vi "Scan Chart View.vi"(10 "UserEvents in":refnum<class "UserEvents.lvclass">) -> ()   [LabVIEW 2015, in "FAMT Views.lvlib"]
uses:
  FAMT Views.lvlib
  UserEvents/UserEvents.lvclass
  UserEvents/UserEvents.lvclass/UserEvents.ctl
  Typedefs/State Types.ctl
  Typedefs/FAMT Typedefs.lvlib
panel:
  out "Chart":cluster{"Current Demand":dbl, dbl}(graph)
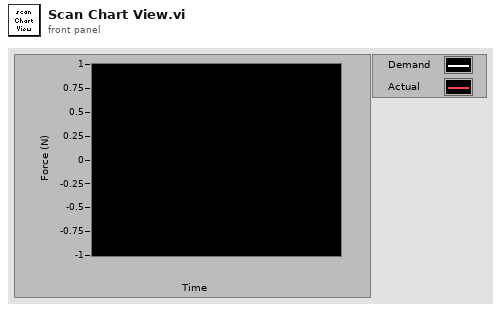
[diagram p1: front panel]
types:
  T1 = typedef "FAMT Typedefs.lvlib/Publish Data Events.ctl" = cluster{"State":refnum<user-event>, "ErrorCode":refnum<user-event>, "FC1 ILC Outputs":refnum<user-event>, "LogPath":refnum<user-event>, "FC1 ILC Inputs":refnum<user-event>, "Scan Progress":refnum<user-event>, "FC2 ILC Outputs":refnum<user-event>, "FC2 ILC Inputs":refnum<user-event>}
  T2 = cluster{"Event Registration Refnum":refnum<event-registration>, "Event Registration Refnum":refnum<event-registration>}
  T3 = typedef "FAMT Typedefs.lvlib/State Types.ctl" = enum16{"Offline State", "Fault State", "Standby State", "Disabled State", "Enabled State", "Wait For User Input State", "Perform Scan State"}
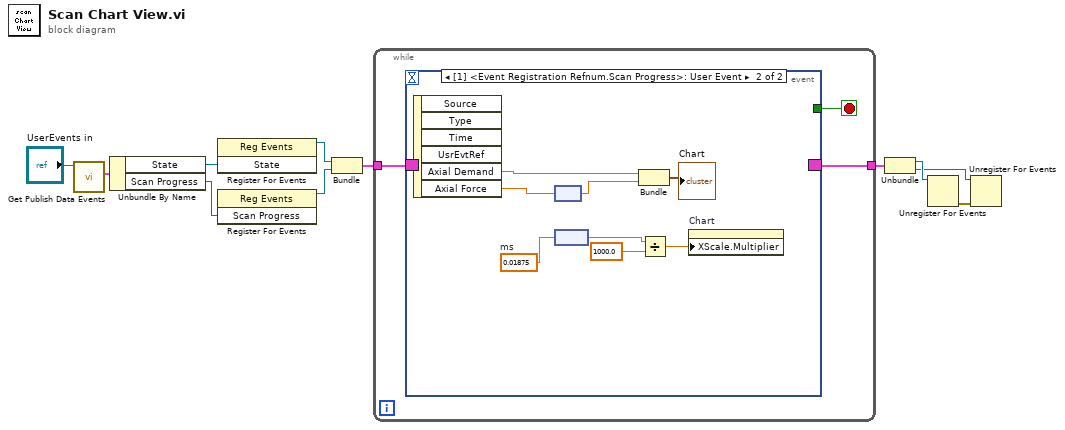
[diagram p0: block diagram]
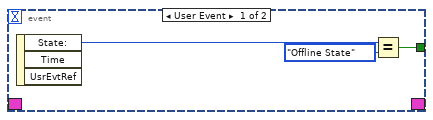
[diagram p2: hidden frame]
diagram:
  n1 = call "Get Publish Data Events.vi"("UserEvents in"="UserEvents in") -> ("Publish Data Events"=w8:T1)  [unwired: 9 in, 1 out]
  n2 = Unbundle By Name(w8) -> ("State"=w9:refnum<user-event>, "Scan Progress"=w7:refnum<user-event>)
  n3 = register-events(w9) -> (reference out=w11:refnum<event-registration>)  [unwired: 2 in, 1 out]
  n4 = register-events(w7) -> (reference out=w10:refnum<event-registration>)  [unwired: 2 in, 1 out]
  n5 = Bundle("Event Registration Refnum"=w11, "Event Registration Refnum"=w10) -> (w3:T2)  [unwired: 1 in]
  n6 = while {
    tunnel: w3 -> [w14]
    tunnel: [w13] -> w2
    stop <- w12 stop-if-true
    n7 = event shown="[1] <Event Registration Refnum.Scan Progress>: User Event" {
      selector: w14 -> [_ _]
      dyn-events: [_ _] -> w13
      timeout: _ -> [_ _]
      tunnel: [w16 _] -> w12
      event User Event {
        n8 = event-data() -> ("State:"=w15:T3)  [unwired: 1 in, 2 out]
        n9 = Equal?(x=w15, y=State_Types."Offline State") -> (x = y?=w16:bool)
      }
      event User Event {
        w19 = dbl[unit] 0.01875  # ms
        n10 = event-data() -> ("Axial Demand"=w20:dbl, "Axial Force"=w25:dbl[unit])  [unwired: 1 in, 4 out]
        n11 = node(w25) -> (w24:dbl)
        n12 = node(w19) -> (w22:dbl)
        n13 = Bundle("Axial Demand"=w20, w24) -> (→"Chart":cluster{"Axial Demand":dbl, dbl})  [unwired: 1 in]
        n14 = Divide(x=w22, y=1000.0) -> (x/y=w21:dbl)
        n15 = property on="Chart" class="WFChart (strict)"("XScale.Multiplier"=w21) -> ()  [unwired: 2 in, 2 out]
      }
    }
  }
  n16 = Unbundle(w2) -> ("Event Registration Refnum"=w6:refnum<event-registration>, "Event Registration Refnum"=w5:refnum<event-registration>)
  n17 = Unregister For Events(event registration refnum=w6) -> (error out=w4:errorcluster)  [unwired: 1 in]
  n18 = Unregister For Events(event registration refnum=w5, error in=w4) -> ()  [unwired: 1 out]
